vi "Configure Frequency and Period.vi"(0 "VISA resource name":refnum<visa-resource-name>, 1 "Scan List (Empty)":string, 5 "Threshold Range (10)":i32=10, 11 "error in (no error)":errorcluster) -> (4 "VISA resource name out":refnum<visa-resource-name>, 15 "error out":errorcluster)   [LabVIEW 2020, in "Keithley 27XX.lvlib"]
doc: "This VI will configure the threshold range for frequency and period measurements.\n\nNote: \n(1) Configure Measurement.vi must be called <B>before</B> setting the threshold range.\n\n(2) This VI will only work in Frequency or Period Measurement modes."
uses:
  <instrlib>/Keithley 27XX/Keithley 27XX.lvlib
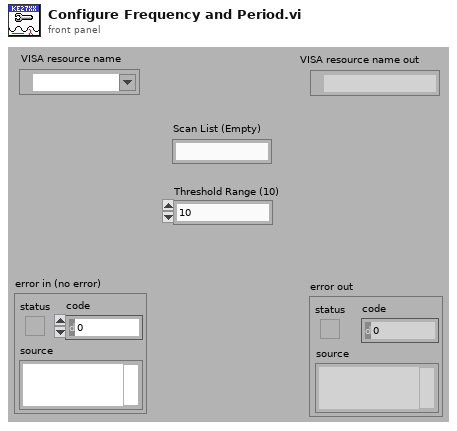
[diagram p1: front panel]
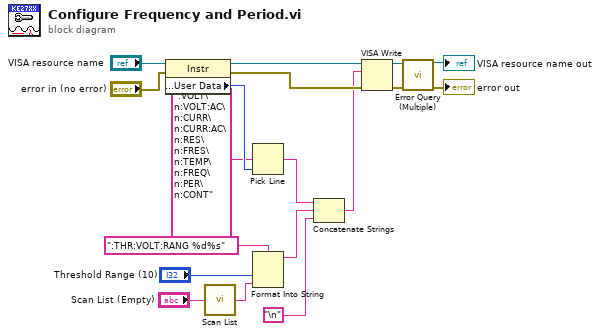
[diagram p0: block diagram]
diagram:
  n1 = property on="Property Node" class="Instr"(reference="VISA resource name", error in="error in (no error)") -> (reference out=w14:refnum<visa-resource-name>, error out=w13:errorcluster, "General Settings:User Data"=w18:u32)
  n2 = call <instrlib>:"Scan List.vi"("Scan List (Empty)"="Scan List (Empty)") -> ("Scan List Out"=w7:string)  [unwired: 14 in]
  n3 = Pick Line(multi-line string=":VOLT\n:VOLT:AC\n:CURR\n:CURR:AC\n:RES\n:FRES\n:TEMP\n:FREQ\n:PER\n:CONT", line index=w18) -> (output string=w12:string)  [unwired: 1 in]
  n4 = Format Into String(format string=":THR:VOLT:RANG %d%s", "Threshold Range (10)", w7) -> (resulting string=w6:string)  [unwired: 2 in, 1 out]
  n5 = Concatenate Strings(w12, w6, "\n") -> (w11:string)
  n6 = VISA Write(VISA resource name=w14, write buffer=w11, error in (no error)=w13) -> (VISA resource name out=w5:refnum<visa-resource-name>, error out=w4:errorcluster)  [unwired: 1 out]
  n7 = call <instrlib>:"Error Query (Multiple).vi"("VISA resource name"=w5, "error in (no error)"=w4) -> ("VISA resource name out"=→"VISA resource name out":refnum<visa-resource-name>, "error out"=→"error out":errorcluster)  [unwired: 10 in, 2 out]
